vi "Format Log to String.vi"(10 "Log Packet":T1, 11 "String Expression Format in":refnum<class "String Expression Format.lvclass">) -> (2 "Log Entry":string, 3 "String Expression Format out":refnum<class "String Expression Format.lvclass">)   [LabVIEW 2019, in "String Expression Format.lvclass"]
uses:
  <vilib>/gpm_packages/@cs/event-logger/Source/String Formats/String Expression Format/String Expression Format.lvclass
  <vilib>/gpm_packages/@cs/event-logger/Source/Composed Log/Types/Log Packet.ctl
  <vilib>/gpm_packages/@cs/event-logger/Source/Composed Log/Types/Log Level.ctl
  <vilib>/gpm_packages/@cs/event-logger/Source/String Formats/String Expression Format/String Expression Format.lvclass/String Expression Format.ctl
  <vilib>/dlg_ctls.llb/Space Constant.vi
  <vilib>/gpm_packages/@cs/event-logger/Source/Composed Log/Composed Log.lvlib
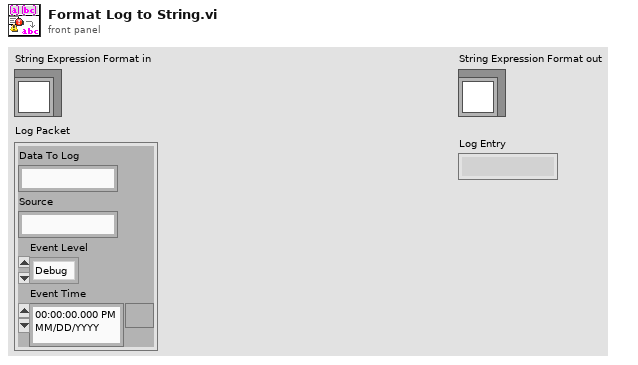
[diagram p1: front panel]
types:
  T1 = typedef "Composed Log.lvlib/Log Packet.ctl" = cluster{"Data To Log":string, "Source":string, "Event Level":T2, "Event Time":timestamp}
  T2 = typedef "Composed Log.lvlib/Log Level.ctl" = enum16{"Debug", "Info", "Warning", "Error", "Critical"}
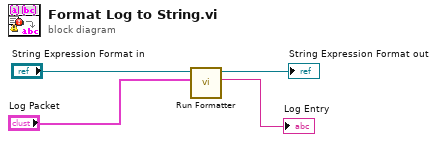
[diagram p0: block diagram]
diagram:
  n1 = call <vilib>:"Run Formatter.vi"("Log Packet"="Log Packet", "String Expression Format in"="String Expression Format in") -> ("Log Entry"=→"Log Entry":string, "String Expression Format out"=→"String Expression Format out":refnum<class "String Expression Format.lvclass">)  [unwired: 7 in, 1 out]
